vi "Write Sub Panel Turnos 1.vi"(8 "error in (no error)":errorcluster, 10 "Sub Panel Turnos":refnum<vi>, 11 "Turnos in":refnum<class "Turnos.lvclass">) -> (0 "error out":errorcluster, 3 "Turnos out":refnum<class "Turnos.lvclass">)   [LabVIEW 2020, in "Turnos.lvlib" / "Turnos.lvclass"]
uses:
  Turnos.lvclass
  Turnos.lvclass/Turnos.ctl
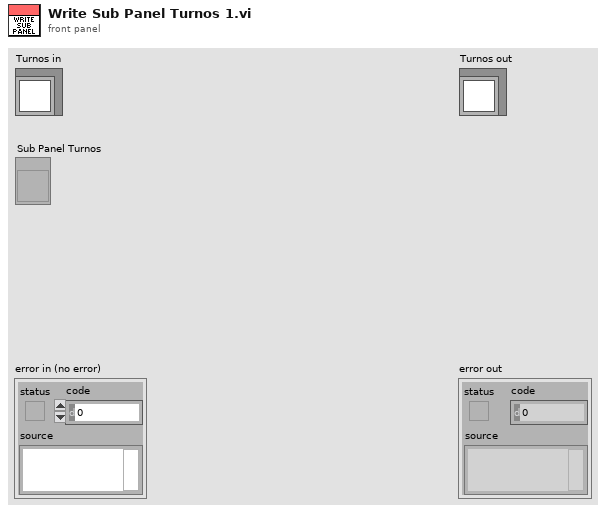
[diagram p1: front panel]
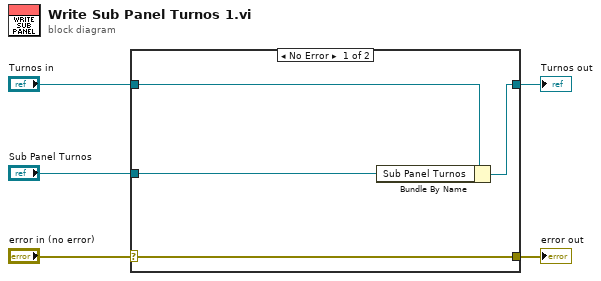
[diagram p0: block diagram]
diagram:
  n1 = case shown="No Error" "error in (no error)" {
    selector: "error in (no error)" -> [w9 w10]
    tunnel: [w9 w10] -> w4
    tunnel: [w7 w11] -> w2
    tunnel: "Turnos in" -> [w8 w11]
    tunnel: "Sub Panel Turnos" -> [w6 _]
    frame No Error {
      n2 = Bundle By Name(cluster=w8, "Sub Panel Turnos"=w6) -> (w7:refnum<class "Turnos.lvclass">)
    }
    frame Error {
    }
  }
  "error out" <- w4
  "Turnos out" <- w2
